vi "rise and fall.vi"(4 "SA data":T1, 6 "Countries":string[](array[string]), 7 "Aggregate indexes":i32[](array[numeric]), 8 "Populations":i32[](array[numeric]), 9 "US data":T1, 10 "deaths CSV":string[][](array[string]), 11 "cases CSV":string[][](array[string])) -> ()   [LabVIEW 2019]
uses:
  Globals.vi
  <vilib>/Utility/config.llb/NI_LVConfig.lvlib
panel:
  in  "Tab Control":enum32{"Results", "Filter out"}(tab)
  in  "Include SA provinces":bool
  in  "How far back to look for rate of rise and fall (days)":u16=14
  in  "Top rate of fall in deaths":i32[](listbox) caption="Top rate of fall in deaths (over last 14 days)"
  in  "Top rate of rise in deaths":i32[](listbox) caption="Top rate of rise in deaths (over last 14 days)"
  in  "Include US states":bool
  in  "Include aggregates":bool
  in  "Aggregates":i32(listbox)
  in  "Remove Button":bool
  in  "Add Button":bool
  in  "Filter out":i32[](listbox)
  in  "Select Country":i32[](listbox)
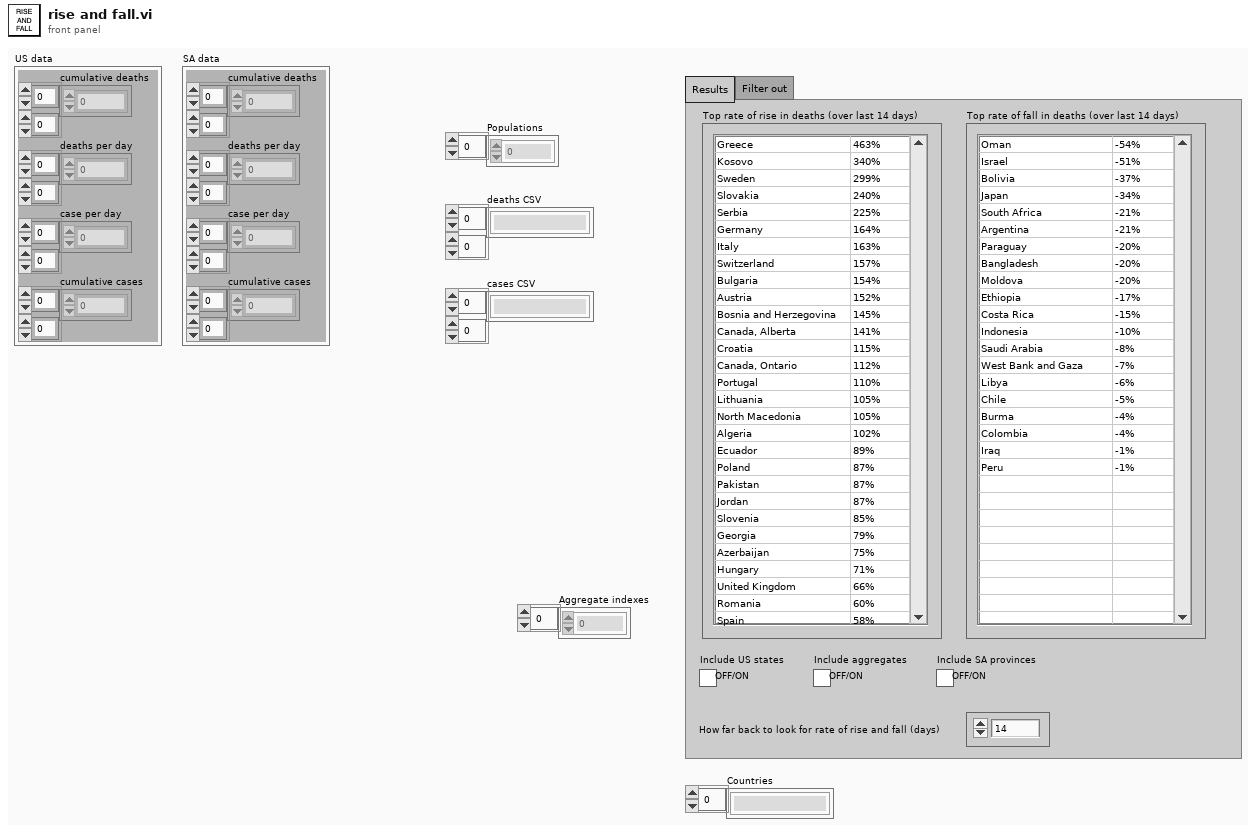
[diagram p1: front panel]
types:
  T1 = cluster{"cumulative deaths":i32[][], "deaths per day":i32[][], "case per day":i32[][], "cumulative cases":i32[][]}
  T2 = typedef "NI_LVConfig.lvlib/Config Data RefNum.ctl" = refnum<k1>
  T3 = cluster{"top new cases":cluster{"country index":i32[], "values":i32[]}, "top new deaths":cluster{"country index":i32[], "values":i32[]}, "top new cases per 1M":cluster{"country index":i32[], "values":dbl[]}, "top new deaths per 1M":cluster{"country index":i32[], "values":dbl[]}, "deaths dropped":cluster{"country index":i32[], "percentage change":dbl[]}, "deaths gained":cluster{"country index":i32[], "percentage change":dbl[]}, "highest deaths per day ever":cluster{"country index":i32[], "highest deaths per day":dbl[]}, "highest deaths":cluster{"country index":i32[], "highest deaths per day":dbl[]}}
  T4 = cluster{"country index":i32[], "percentage change":dbl[]}
  T5 = cluster{"country index":i32[], "highest deaths per day":dbl[]}
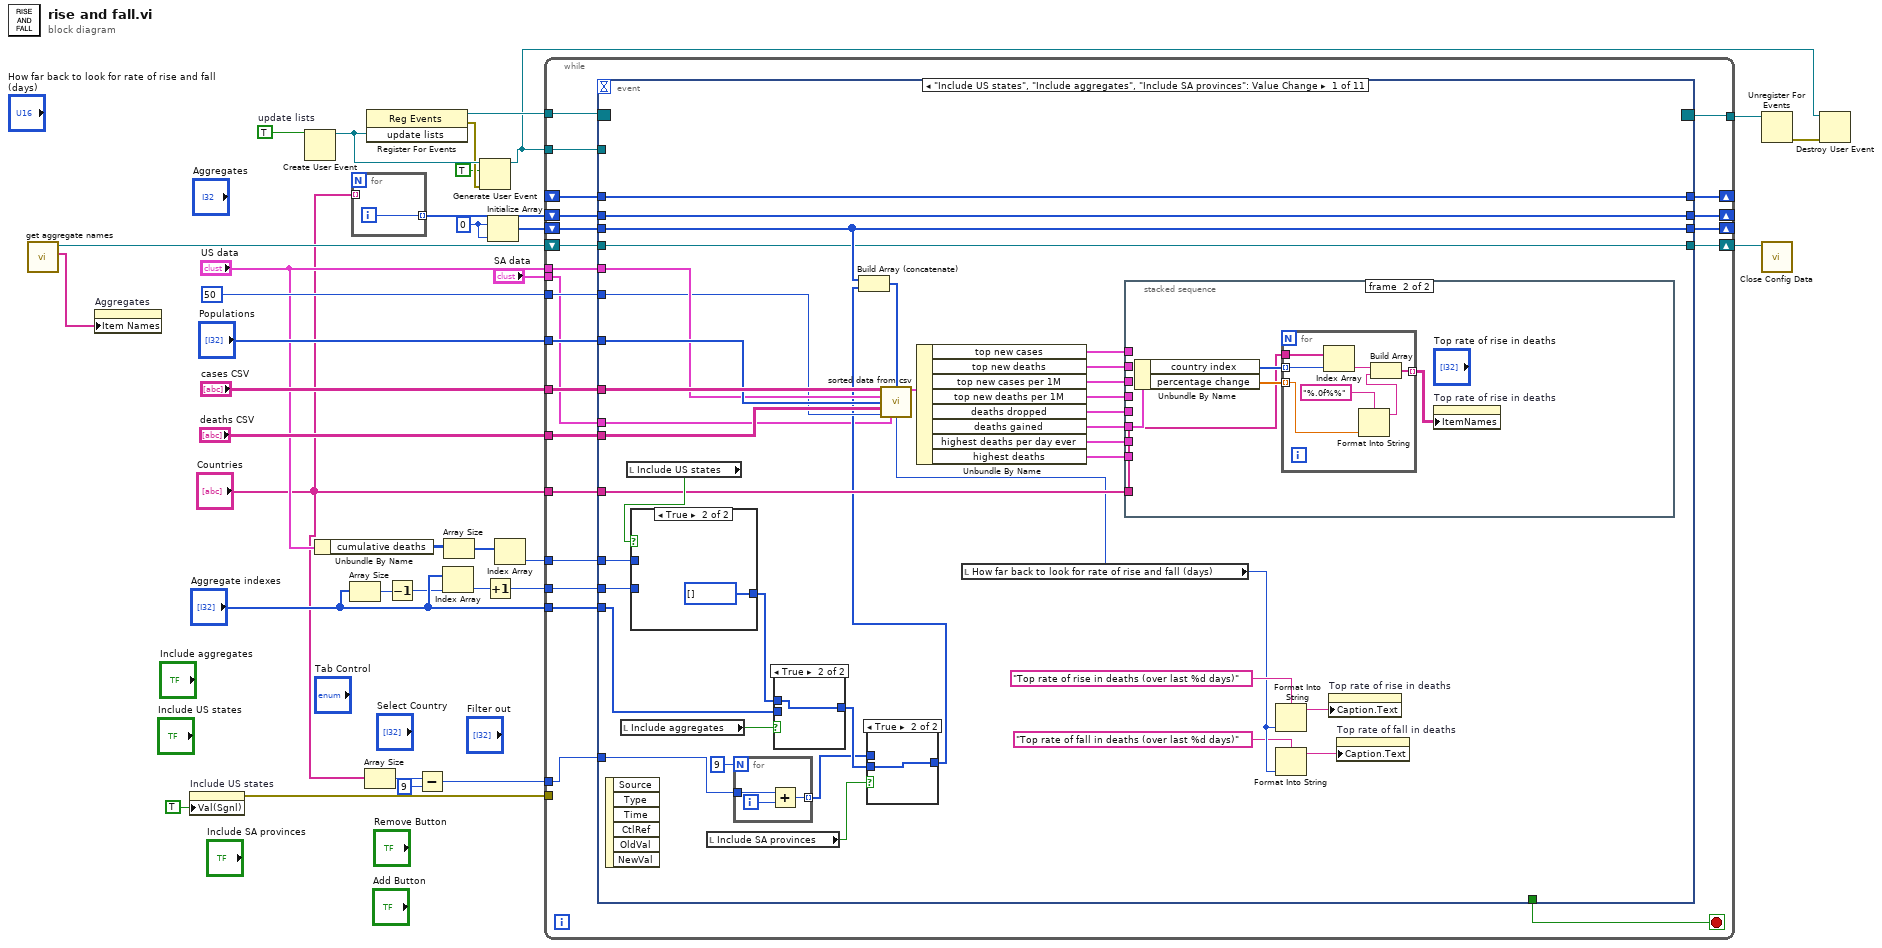
[diagram p0: block diagram]
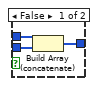
[diagram p2: hidden frame]
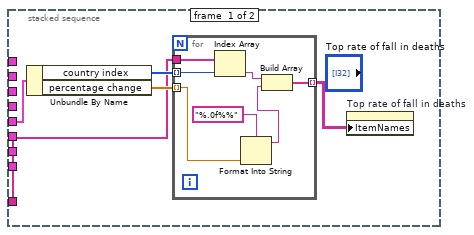
[diagram p3: hidden frame]
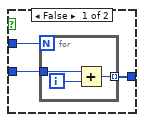
[diagram p4: hidden frame]
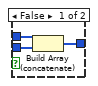
[diagram p5: hidden frame]
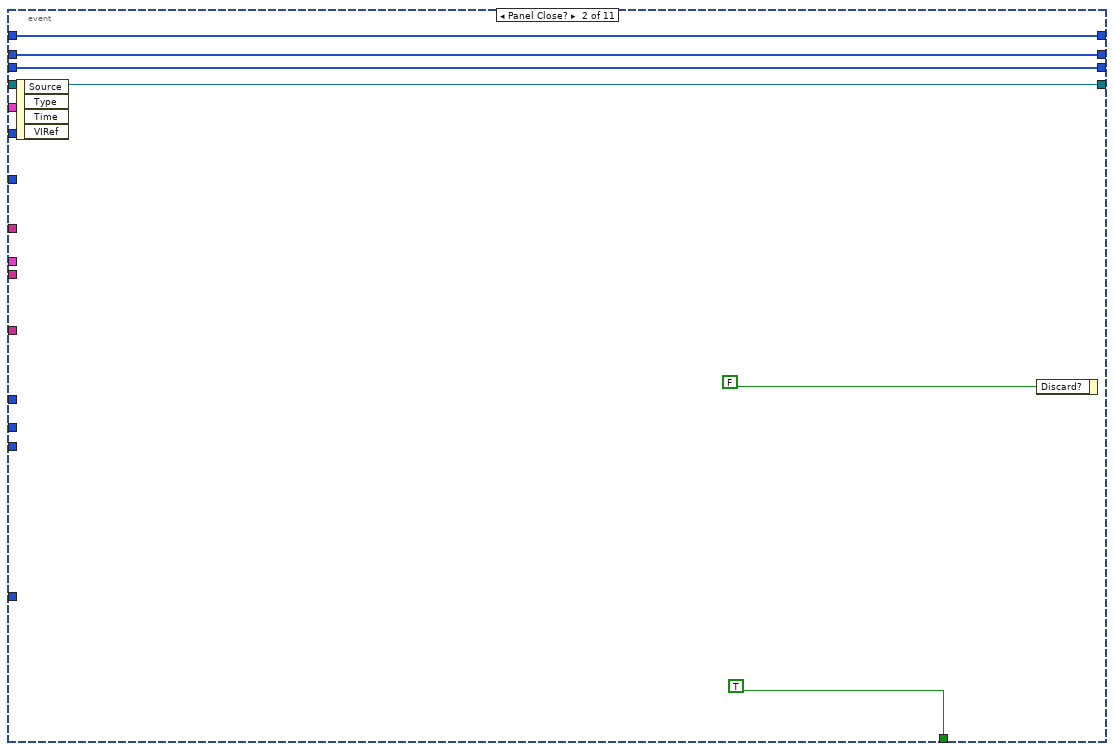
[diagram p6: hidden frame]
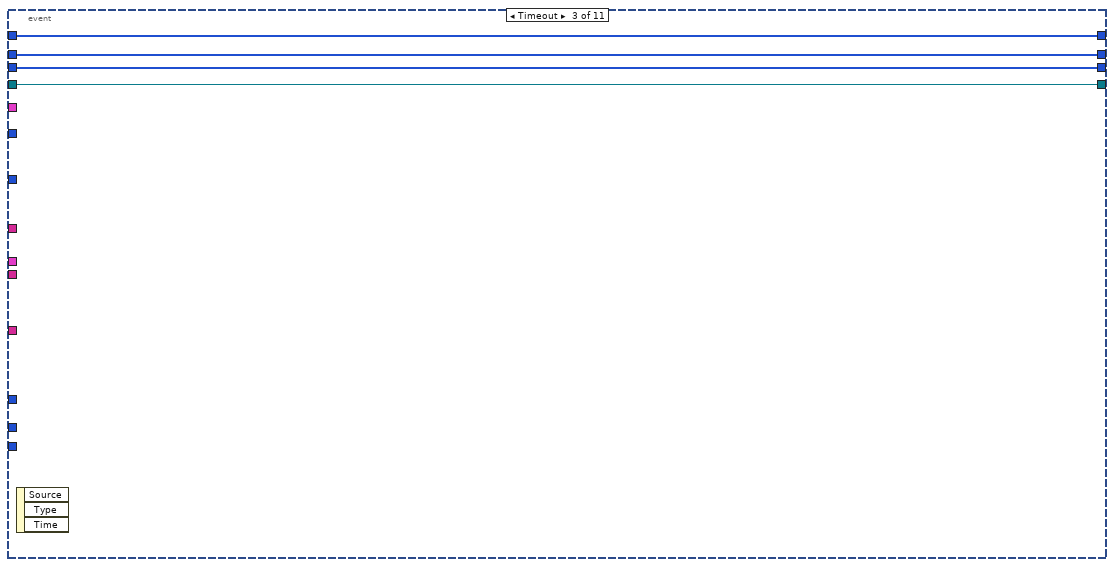
[diagram p7: hidden frame]
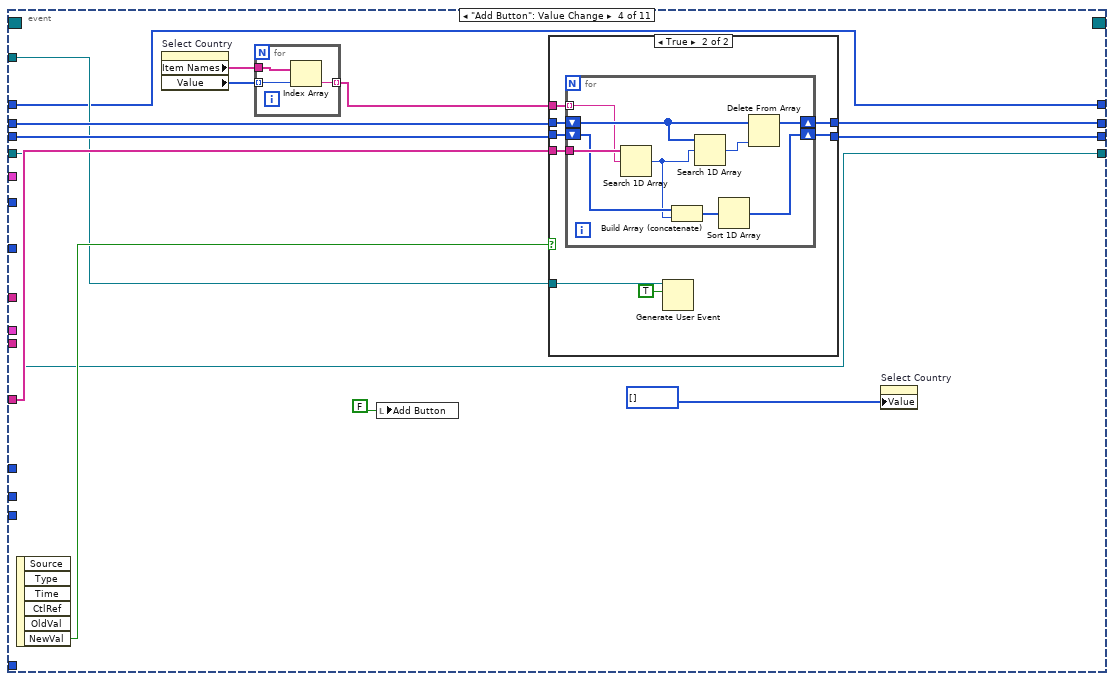
[diagram p8: hidden frame]
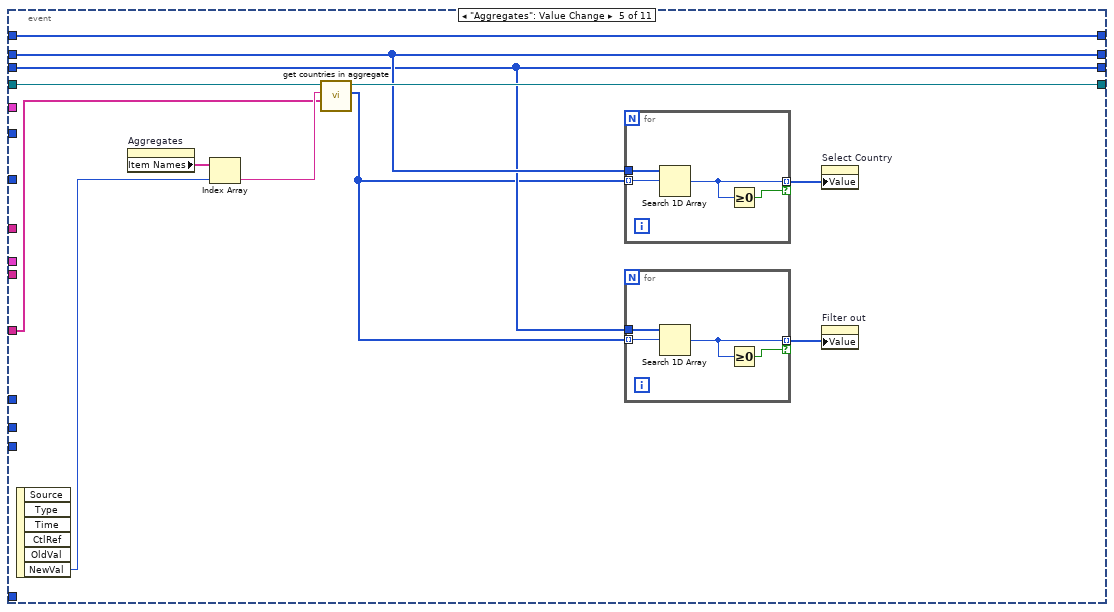
[diagram p10: hidden frame]
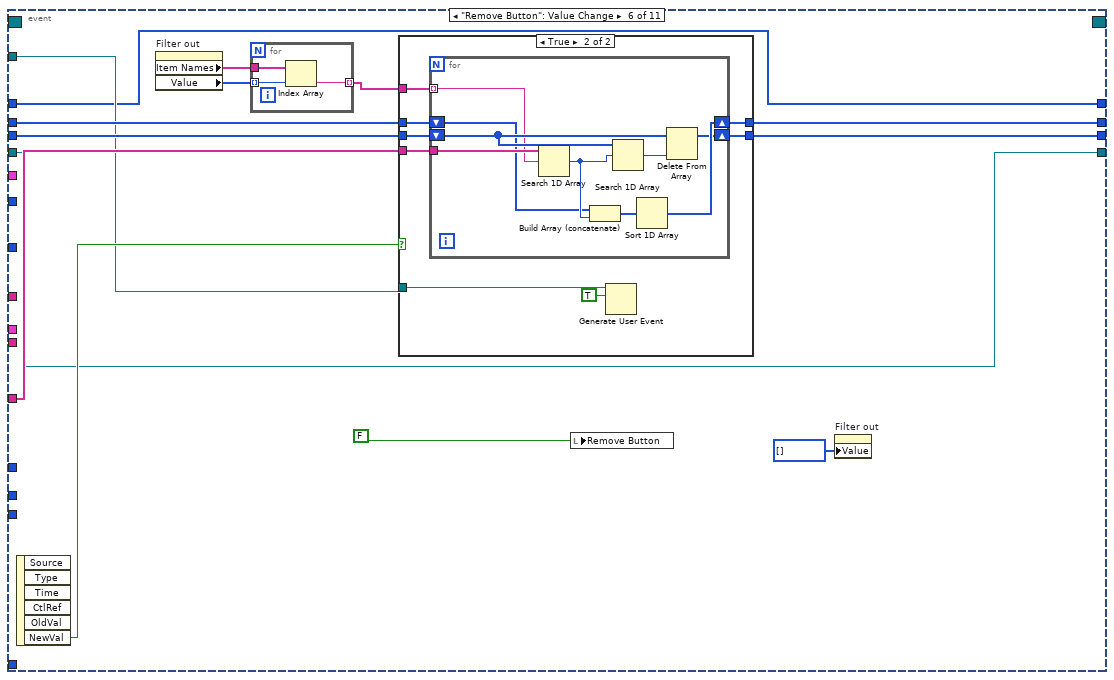
[diagram p11: hidden frame]
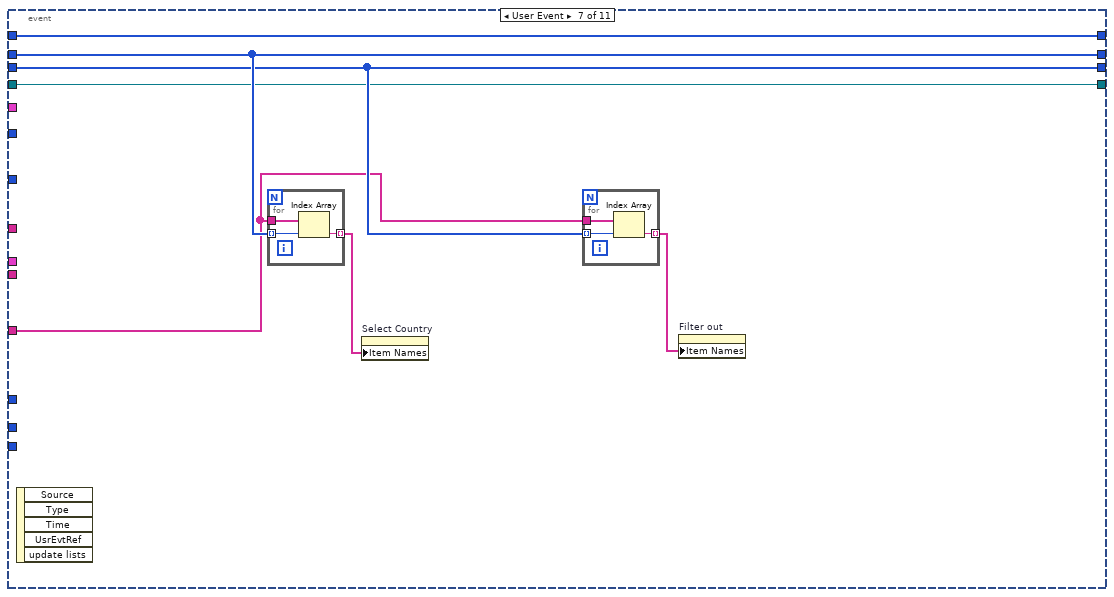
[diagram p13: hidden frame]
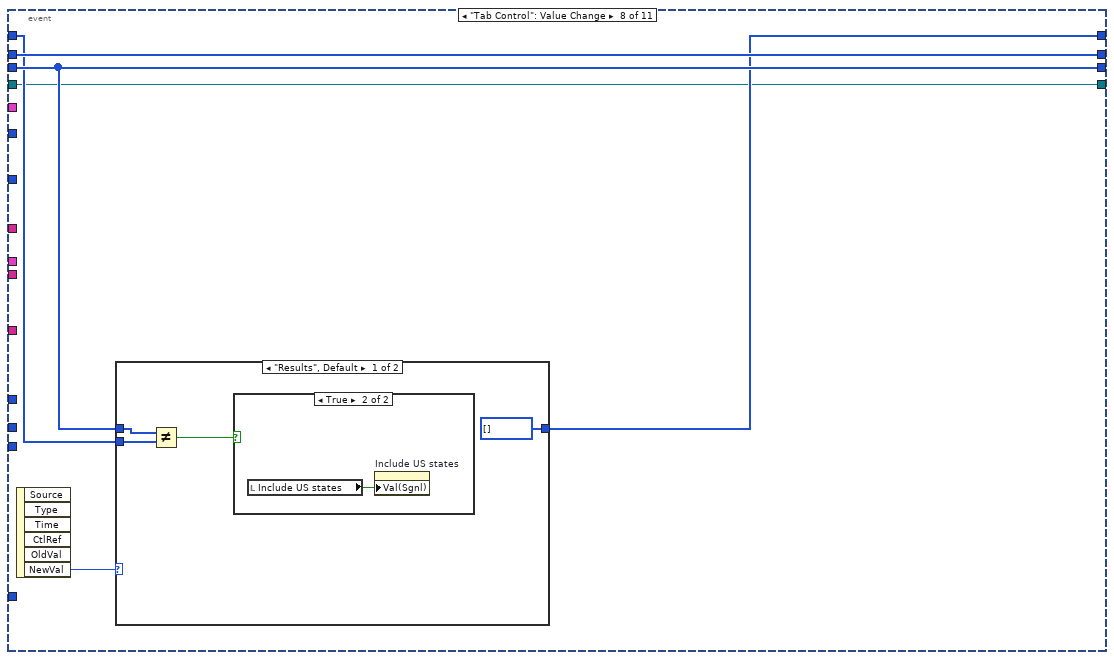
[diagram p14: hidden frame]
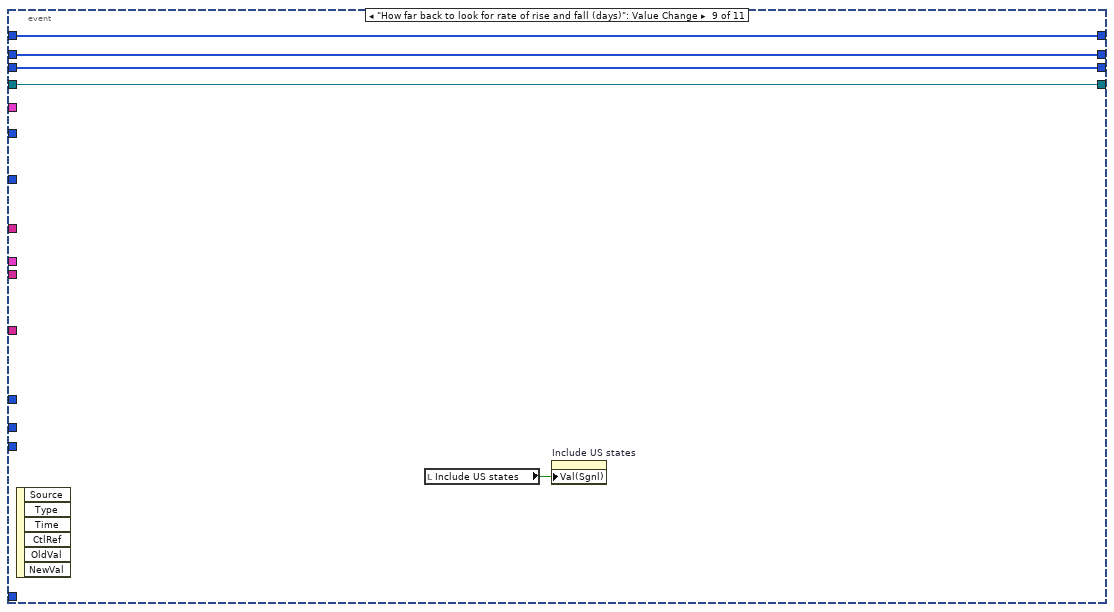
[diagram p17: hidden frame]
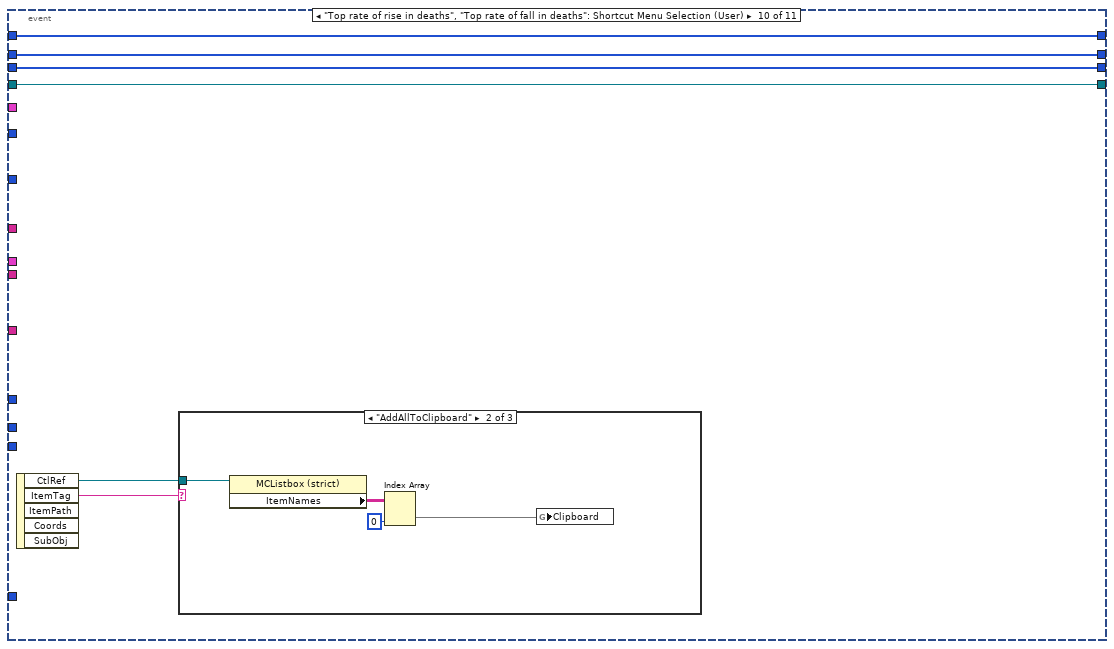
[diagram p18: hidden frame]
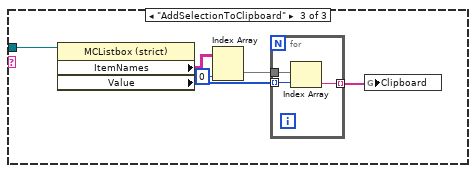
[diagram p20: hidden frame]
diagram:
  w19 = TRUE  # update lists
  w22 = 0
  n1 = call "get aggregate names.vi"() -> ("section names"=w8:string[], "Refnum out"=w7:T2)  [unwired: 10 in]
  n2 = property on="Aggregates" class="LstBox (strict)"("Item Names"=w8) -> ()  [unwired: 2 in, 2 out]
  n3 = property on="Include US states" class="Bool (strict)"("Val(Sgnl)"=TRUE ("Value (Signaling)")) -> (error out=w29:errorcluster)  [unwired: 2 in, 1 out]
  n4 = Create User Event(user event datatype=w19) -> (user event=w15:refnum<user-event>)  [unwired: 1 in, 1 out]
  n5 = Unbundle By Name("US data") -> ("cumulative deaths"=w27:i32[][])
  n6 = Array Size(array="Aggregate indexes") -> (size(s)=w10:i32)
  n7 = for {
    tunnel: "Countries" -> [_] mode=indexing
    tunnel: [w35] -> w20 mode=indexing
    i -> [w35]
  }
  n8 = Array Size(array="Countries") -> (size(s)=w4:i32)
  n9 = register-events(w15) -> (reference out=w18:refnum<event-registration>, error out=w13:errorcluster)  [unwired: 2 in]
  n10 = Decrement(x=w10) -> (x-1=w9:i32)
  n11 = Subtract(x=w4, y=9) -> (x-y=w2:i32)
  n12 = Index Array(array="Aggregate indexes", index=w9) -> (element=w24:i32)
  n13 = Array Size(array=w27) -> (size(s)=w26:i32[])
  n14 = Generate User Event(user event=w15, event data cluster=TRUE ("event data"), error in=w13) -> (user event out=w14:refnum<user-event>)  [unwired: 1 in, 1 out]
  n15 = Increment(x=w24) -> (x+1=w23:i32)
  n16 = Initialize Array(w22, w22) -> (w21:i32[])
  n17 = Index Array(array=w26) -> (element=w25:i32)  [unwired: 1 in]
  n18 = while {
    tunnel: "cases CSV" -> [w58]
    tunnel: "deaths CSV" -> [w57]
    tunnel: "Countries" -> [w56]
    tunnel: "Populations" -> [w55]
    tunnel: "US data" -> [w54]
    tunnel: 50 ("top selection") -> [w53]
    tunnel: w29 -> [_]
    tunnel: "Aggregate indexes" -> [w51]
    tunnel: w25 -> [w50]
    tunnel: w23 -> [w49]
    shift-right: [w47] -> _
    shift-left: w20 -> [w48]
    shift-right: [w45] -> _
    shift-left: w21 -> [w46]
    tunnel: w18 -> [w44]
    tunnel: w14 -> [w43]
    tunnel: [w42] -> w17
    shift-right: [w41] -> _
    shift-left: _ -> [w40]
    shift-right: [w38] -> w6
    shift-left: w7 -> [w39]
    tunnel: w2 -> [w37]
    tunnel: "SA data" -> [w36]
    stop <- w52 stop-if-true
    n19 = event shown="[0] \"Include US states\", \"Include aggregates\", \"Include SA provinces\": Value Change" {
      selector: w44 -> [_ _ _ _ _ _ _ _ _ _ _]
      dyn-events: [_ _ _ _ _ _ _ _ _ _ _] -> w42
      timeout: _ -> [_ _ _ _ _ _ _ _ _ _ _]
      tunnel: w58 -> [w96 _ _ _ _ _ _ _ _ _ _]
      tunnel: w57 -> [w95 _ _ _ _ _ _ _ _ _ _]
      tunnel: w56 -> [w78 _ _ w160 w191 w214 w245 _ _ _ w292]
      tunnel: w55 -> [w94 _ _ _ _ _ _ _ _ _ _]
      tunnel: w54 -> [w93 _ _ _ _ _ _ _ _ _ _]
      tunnel: w53 -> [w92 _ _ _ _ _ _ _ _ _ _]
      tunnel: [_ TRUE _ _ _ _ _ _ _ _ _] -> w52
      tunnel: w51 -> [w90 _ _ _ _ _ _ _ _ _ _]
      tunnel: w50 -> [w87 _ _ _ _ _ _ _ _ _ _]
      tunnel: w49 -> [w86 _ _ _ _ _ _ _ _ _ _]
      tunnel: w48 -> [w85 w142 w148 w162 w190 w218 w247 w259 w270 w276 w300]
      tunnel: [w85 w142 w148 w159 w190 w216 w247 w259 w270 w276 w296] -> w47
      tunnel: w46 -> [w83 w141 w147 w161 w186 w217 w246 w257 w269 w275 w299]
      tunnel: [w83 w141 w147 w158 w186 w215 w246 w257 w269 w275 w295] -> w45
      tunnel: w43 -> [_ _ _ w156 _ w212 _ _ _ _ w290]
      tunnel: [w82 w140 w146 w155 w196 w211 w242 w256 w268 w274 w297] -> w41
      tunnel: w40 -> [w82 w140 w146 w155 w196 w211 w242 w255 w268 w274 w301]
      tunnel: w39 -> [w81 w139 w145 w151 w195 w210 w241 w254 w267 w273 w298]
      tunnel: [w81 w139 w145 w151 w194 w210 w241 w254 w267 w273 w294] -> w38
      tunnel: w37 -> [w60 _ _ _ _ _ _ _ _ _ _]
      tunnel: w36 -> [w59 _ _ _ _ _ _ _ _ _ _]
      event "Include US states", "Include aggregates", "Include SA provinces": Value Change {
        n20 = event-data() -> ()  [unwired: 1 in, 6 out]
        n21 = local read "Include aggregates"() -> (w91:bool)
        n22 = local read "Include US states"() -> (w89:bool)
        n23 = case shown="True" w89 {
          tunnel: [w130 i32[] [] ("Aggregate indexes")] -> w88
          tunnel: w87 -> [w129 _]
          tunnel: w86 -> [w128 _]
          frame False {
            n24 = for {
              N: w129 -> [_]
              tunnel: [w133] -> w130 mode=indexing
              tunnel: w128 -> [w131]
              i -> [w132]
              n25 = Add(x=w131, y=w132) -> (x+y=w133:i32)
            }
          }
          frame True {
          }
        }
        n26 = local read "Include SA provinces"() -> (w64:bool)
        n27 = for {
          N: 9 -> [_]
          tunnel: [w99] -> w61 mode=indexing
          tunnel: w60 -> [w97]
          i -> [w98]
          n28 = Add(x=w97, y=w98) -> (x+y=w99:i32)
        }
        n29 = case shown="True" w91 {
          tunnel: w90 -> [w137 _]
          tunnel: [w136 w138] -> w63
          tunnel: w88 -> [w135 w138]
          frame False {
            n30 = Build Array (concatenate)(w135, w137) -> (w136:i32[])
          }
          frame True {
          }
        }
        n31 = case shown="True" w64 {
          tunnel: w63 -> [w102 w103]
          tunnel: [w101 w103] -> w65
          tunnel: w61 -> [w100 _]
          frame False {
            n32 = Build Array (concatenate)(w100, w102) -> (w101:i32[])
          }
          frame True {
          }
        }
        n33 = Build Array (concatenate)(w83, w65) -> (w84:i32[])
        n34 = local read "How far back to look for rate of rise and fall (days)"() -> (w69:u16)
        n35 = call "sorted data from csv.vi"("cases CSV"=w96, "filter out"=w84, "US data"=w93, "Populations"=w94, "deaths CSV"=w95, "top selection"=w92, "SA data"=w59, "period in days to check"=w69) -> ("ranked results"=w80:T3)  [unwired: 7 in]
        n36 = Unbundle By Name(w80) -> ("top new cases"=w79:cluster{"country index":i32[], "values":i32[]}, "top new deaths"=w77:cluster{"country index":i32[], "values":i32[]}, "top new cases per 1M"=w76:cluster{"country index":i32[], "values":dbl[]}, "top new deaths per 1M"=w75:cluster{"country index":i32[], "values":dbl[]}, "deaths dropped"=w74:T4, "deaths gained"=w73:T4, "highest deaths per day ever"=w72:T5, "highest deaths"=w71:T5)
        n37 = stacked-sequence {
          tunnel: w79 -> [_ _]
          tunnel: w78 -> [w105 w117]
          tunnel: w77 -> [_ _]
          tunnel: w76 -> [_ _]
          tunnel: w75 -> [_ _]
          tunnel: w74 -> [w106 _]
          tunnel: w73 -> [_ w118]
          tunnel: w72 -> [_ _]
          tunnel: w71 -> [_ _]
          frame #0 {
            n38 = Unbundle By Name(w106) -> ("country index"=w107:i32[], "percentage change"=w108:dbl[])
            n39 = for {
              tunnel: w107 -> [w114] mode=indexing
              tunnel: w105 -> [w115]
              tunnel: w108 -> [w110] mode=indexing
              tunnel: [w112] -> w104 mode=indexing
              n40 = Index Array(array=w115, index=w114) -> (element=w113:string)
              n41 = Format Into String(format string="%.0f%%", w110) -> (resulting string=w109:string)  [unwired: 2 in, 1 out]
              n42 = Build Array(w113, w109) -> (w112:string[])
            }
            n43 = property on="Top rate of fall in deaths" class="MCListbox (strict)"("ItemNames"=w104) -> ()  [unwired: 2 in, 2 out]
          }
          frame #1 {
            n44 = Unbundle By Name(w118) -> ("country index"=w119:i32[], "percentage change"=w120:dbl[])
            n45 = for {
              tunnel: w119 -> [w126] mode=indexing
              tunnel: w117 -> [w127]
              tunnel: w120 -> [w122] mode=indexing
              tunnel: [w124] -> w116 mode=indexing
              n46 = Index Array(array=w127, index=w126) -> (element=w125:string)
              n47 = Format Into String(format string="%.0f%%", w122) -> (resulting string=w121:string)  [unwired: 2 in, 1 out]
              n48 = Build Array(w125, w121) -> (w124:string[])
            }
            n49 = property on="Top rate of rise in deaths" class="MCListbox (strict)"("ItemNames"=w116) -> ()  [unwired: 2 in, 2 out]
          }
        }
        n50 = Format Into String(format string="Top rate of rise in deaths (over last %d days)", w69) -> (resulting string=w68:string)  [unwired: 2 in, 1 out]
        n51 = Format Into String(format string="Top rate of fall in deaths (over last %d days)", w69) -> (resulting string=w67:string)  [unwired: 2 in, 1 out]
        n52 = property on="Top rate of rise in deaths" class="MCListbox (strict)"("Caption.Text"=w68) -> ()  [unwired: 2 in, 2 out]
        n53 = property on="Top rate of fall in deaths" class="MCListbox (strict)"("Caption.Text"=w67) -> ()  [unwired: 2 in, 2 out]
      }
      event Panel Close? {
        n54 = event-data() -> ()  [unwired: 1 in, 4 out]
        n55 = event-data("Discard?"=FALSE) -> ()  [unwired: 1 in, 1 out]
      }
      event Timeout {
        n56 = event-data() -> ()  [unwired: 1 in, 3 out]
      }
      event "Add Button": Value Change {
        n57 = event-data() -> ("NewVal"=w157:bool)  [unwired: 1 in, 5 out]
        n58 = property on="Select Country" class="LstBox (strict)"() -> ("Item Names"=w153:string[], "Value"=w154:i32[])  [unwired: 2 in, 2 out]
        n59 = for {
          tunnel: w154 -> [w165] mode=indexing
          tunnel: w153 -> [w164]
          tunnel: [w163] -> w152 mode=indexing
          n60 = Index Array(array=w164, index=w165) -> (element=w163:string)
        }
        n61 = local write "Add Button"(FALSE ("Add Button")) -> ()
        n62 = case shown="True" w157 {
          tunnel: w162 -> [w167 w174]
          tunnel: w160 -> [_ w175]
          tunnel: [w167 w169] -> w159
          tunnel: w161 -> [w166 w173]
          tunnel: [w166 w170] -> w158
          tunnel: w156 -> [_ w172]
          tunnel: w152 -> [_ w168]
          frame False {
          }
          frame True {
            n63 = for {
              tunnel: w175 -> [w184]
              shift-right: [w178] -> w170
              shift-left: w173 -> [w181]
              shift-right: [w177] -> w169
              shift-left: w174 -> [w182]
              tunnel: w168 -> [w176] mode=indexing
              n64 = Search 1D Array(1D array=w184, element=w176) -> (index of element=w180:i32)  [unwired: 1 in]
              n65 = Build Array (concatenate)(w181, w180) -> (w179:i32[])
              n66 = Search 1D Array(1D array=w182, element=w180) -> (index of element=w183:i32)  [unwired: 1 in]
              n67 = Sort 1D Array(array=w179) -> (sorted array=w178:i32[])
              n68 = Delete From Array(array=w182, index=w183) -> (array with subset deleted=w177:i32[])  [unwired: 1 in, 1 out]
            }
            n69 = Generate User Event(user event=w172, event data cluster=TRUE ("event data")) -> ()  [unwired: 2 in, 2 out]
          }
        }
        n70 = property on="Select Country" class="LstBox (strict)"("Value"=i32[] [] ("Select Country")) -> ()  [unwired: 2 in, 2 out]
      }
      event "Aggregates": Value Change {
        n71 = event-data() -> ("NewVal"=w188:i32)  [unwired: 1 in, 5 out]
        n72 = property on="Aggregates" class="LstBox (strict)"() -> ("Item Names"=w193:string[])  [unwired: 2 in, 2 out]
        n73 = Index Array(array=w193, index=w188) -> (element=w192:string)
        n74 = call "get countries in aggregate.vi"("countries"=w191, "aggregate name"=w192, "Refnum in"=w195) -> ("country indexes"=w185:i32[], "Refnum out"=w194:T2)  [unwired: 7 in]
        n75 = for {
          tunnel: w185 -> [w204] mode=indexing
          tunnel: w190 -> [w203]
          tunnel: [w202] -> w189 mode=indexing if=w201
          n76 = Search 1D Array(1D array=w203, element=w204) -> (index of element=w202:i32)  [unwired: 1 in]
          n77 = Greater Or Equal To 0?(x=w202) -> (x >= 0?=w201:bool)
        }
        n78 = for {
          tunnel: w185 -> [w200] mode=indexing
          tunnel: w186 -> [w199]
          tunnel: [w198] -> w187 mode=indexing if=w197
          n79 = Search 1D Array(1D array=w199, element=w200) -> (index of element=w198:i32)  [unwired: 1 in]
          n80 = Greater Or Equal To 0?(x=w198) -> (x >= 0?=w197:bool)
        }
        n81 = property on="Select Country" class="LstBox (strict)"("Value"=w189) -> ()  [unwired: 2 in, 2 out]
        n82 = property on="Filter out" class="LstBox (strict)"("Value"=w187) -> ()  [unwired: 2 in, 2 out]
      }
      event "Remove Button": Value Change {
        n83 = event-data() -> ("NewVal"=w213:bool)  [unwired: 1 in, 5 out]
        n84 = property on="Filter out" class="LstBox (strict)"() -> ("Item Names"=w207:string[], "Value"=w206:i32[])  [unwired: 2 in, 2 out]
        n85 = for {
          tunnel: w207 -> [w221]
          tunnel: w206 -> [w220] mode=indexing
          tunnel: [w219] -> w205 mode=indexing
          n86 = Index Array(array=w221, index=w220) -> (element=w219:string)
        }
        n87 = case shown="True" w213 {
          tunnel: w218 -> [w223 w229]
          tunnel: w214 -> [_ w231]
          tunnel: [w223 w225] -> w216
          tunnel: w217 -> [w222 w230]
          tunnel: [w222 w224] -> w215
          tunnel: w212 -> [_ w228]
          tunnel: w205 -> [_ w226]
          frame False {
          }
          frame True {
            n88 = for {
              tunnel: w231 -> [w240]
              tunnel: w226 -> [w234] mode=indexing
              shift-right: [w233] -> w225
              shift-left: w229 -> [w235]
              shift-right: [w232] -> w224
              shift-left: w230 -> [w236]
              n89 = Search 1D Array(1D array=w240, element=w234) -> (index of element=w238:i32)  [unwired: 1 in]
              n90 = Build Array (concatenate)(w235, w238) -> (w237:i32[])
              n91 = Search 1D Array(1D array=w236, element=w238) -> (index of element=w239:i32)  [unwired: 1 in]
              n92 = Sort 1D Array(array=w237) -> (sorted array=w233:i32[])
              n93 = Delete From Array(array=w236, index=w239) -> (array with subset deleted=w232:i32[])  [unwired: 1 in, 1 out]
            }
            n94 = Generate User Event(user event=w228, event data cluster=TRUE ("event data")) -> ()  [unwired: 2 in, 2 out]
          }
        }
        n95 = local write "Remove Button"(FALSE ("Remove Button")) -> ()
        n96 = property on="Filter out" class="LstBox (strict)"("Value"=i32[] [] ("Filter out")) -> ()  [unwired: 2 in, 2 out]
      }
      event User Event {
        n97 = event-data() -> ()  [unwired: 1 in, 5 out]
        n98 = for {
          tunnel: w247 -> [w252] mode=indexing
          tunnel: w245 -> [w253]
          tunnel: [w251] -> w244 mode=indexing
          n99 = Index Array(array=w253, index=w252) -> (element=w251:string)
        }
        n100 = property on="Select Country" class="LstBox (strict)"("Item Names"=w244) -> ()  [unwired: 2 in, 2 out]
        n101 = for {
          tunnel: w246 -> [w249] mode=indexing
          tunnel: w245 -> [w250]
          tunnel: [w248] -> w243 mode=indexing
          n102 = Index Array(array=w250, index=w249) -> (element=w248:string)
        }
        n103 = property on="Filter out" class="LstBox (strict)"("Item Names"=w243) -> ()  [unwired: 2 in, 2 out]
      }
      event "Tab Control": Value Change {
        n104 = event-data() -> ("NewVal"=w258:enum32{"Results", "Filter out"})  [unwired: 1 in, 5 out]
        n105 = case shown="\"Results\", Default" w258 {
          tunnel: w257 -> [w263 w265]
          tunnel: [i32[] [] w265] -> w256
          tunnel: w255 -> [w262 _]
          frame "Results", Default {
            n106 = Not Equal?(x=w263, y=w262) -> (x != y?=w260:bool)
            n107 = case shown="True" w260 {
              frame False {
              }
              frame True {
                n108 = local read "Include US states"() -> (w264:bool)
                n109 = property on="Include US states" class="Bool (strict)"("Val(Sgnl)"=w264) -> ()  [unwired: 2 in, 2 out]
              }
            }
          }
          frame "Filter out" {
          }
        }
      }
      event "How far back to look for rate of rise and fall (days)": Value Change {
        n110 = event-data() -> ()  [unwired: 1 in, 6 out]
        n111 = local read "Include US states"() -> (w266:bool)
        n112 = property on="Include US states" class="Bool (strict)"("Val(Sgnl)"=w266) -> ()  [unwired: 2 in, 2 out]
      }
      event "Top rate of rise in deaths", "Top rate of fall in deaths": Shortcut Menu Selection (User) {
        n113 = event-data() -> ("CtlRef"=w271:refnum<vi>, "ItemTag"=w272:string)  [unwired: 1 in, 3 out]
        n114 = case shown="\"AddAllToClipboard\"" w272 {
          tunnel: w271 -> [_ w278 w286]
          frame "False", Default {
          }
          frame "AddAllToClipboard" {
            n115 = property class="MCListbox (strict)"(reference=w278) -> ("ItemNames"=w280:string[][])  [unwired: 1 in, 2 out]
            n116 = Index Array(array=w280, index (col)=0 ("disabled index (col)")) -> (element=w277:string[])  [unwired: 1 in]
            n117 = global write "Globals.vi" "Clipboard"(w277) -> ()
          }
          frame "AddSelectionToClipboard" {
            n118 = property class="MCListbox (strict)"(reference=w286) -> ("ItemNames"=w284:string[][], "Value"=w285:i32[])  [unwired: 1 in, 2 out]
            n119 = Index Array(array=w284, index (col)=0 ("disabled index (col)")) -> (element=w282:string[])  [unwired: 1 in]
            n120 = for {
              tunnel: w285 -> [w289] mode=indexing
              tunnel: w282 -> [w288]
              tunnel: [w287] -> w281 mode=indexing
              n121 = Index Array(array=w288, index=w289) -> (element=w287:string)
            }
            n122 = global write "Globals.vi" "Clipboard"(w281) -> ()
          }
        }
      }
      event "Aggregates": Shortcut Menu Selection (User) {
        n123 = event-data() -> ("CtlRef"=w291:refnum<vi>, "ItemTag"=w293:string)  [unwired: 1 in, 6 out]
        n124 = case shown="\"Filter_out_all_except_selection\"" w293 {
          tunnel: w301 -> [w313 w319]
          tunnel: w300 -> [_ w318]
          tunnel: w299 -> [_ w317]
          tunnel: w298 -> [w309 w316]
          tunnel: [w313 w319] -> w297
          tunnel: [w310 w318] -> w296
          tunnel: [w311 w317] -> w295
          tunnel: [w309 w316] -> w294
          tunnel: w292 -> [w314 _]
          tunnel: w291 -> [_ _]
          tunnel: w290 -> [w305 _]
          frame "Filter_out_all_except_selection" {
            w312 = 0
            n125 = Initialize Array(w312, w312) -> (w310:i32[])
            n126 = for {
              tunnel: [w315] -> w311 mode=indexing
              tunnel: w314 -> [_] mode=indexing
              i -> [w315]
            }
            n127 = property on="Aggregates" class="LstBox (strict)"() -> (error out=w306:errorcluster, "Value"=w307:i32)  [unwired: 2 in, 1 out]
            n128 = property on="Aggregates" class="LstBox (strict)"(error in=w306, "Val(Sgnl)"=w307) -> (error out=w303:errorcluster)  [unwired: 1 in, 1 out]
            n129 = Generate User Event(user event=w305, event data cluster=TRUE ("event data"), error in=w303) -> (error out=w302:errorcluster)  [unwired: 1 in, 1 out]
            n130 = property on="Remove Button" class="Bool (strict)"(error in=w302, "Val(Sgnl)"=TRUE ("Value (Signaling)")) -> ()  [unwired: 1 in, 2 out]
          }
          frame "True", Default {
          }
        }
      }
    }
  }
  n131 = Unregister For Events(event registration refnum=w17) -> (error out=w16:errorcluster)  [unwired: 1 in]
  n132 = call <vilib>:"Close Config Data.vi"("refnum"=w6) -> ()  [unwired: 9 in, 2 out]
  n133 = Destroy User Event(user event=w14, error in=w16) -> ()  [unwired: 1 out]
